vi "Confirm Delays.vi"(3 "Modes":cluster{"A=":u16, "B=":u16, "C=":u16, "D=":u16} {"D=" items=["T0+", "A+", "B+", "C+"]; "C=" items=["T0+", "A+", "B+", "D+"]; "B=" items=["T0+", "A+", "C+", "D+"]; "A=" items=["T0+", "B+", "C+", "D+"]}, 5 "Delays (s)":dbl[](array[numeric]) min=0.0 max=1000.0 format="%#_15f") -> (0 "Modes (out)":cluster{"A=":u16, "B=":u16, "C=":u16, "D=":u16} {"D=" items=["T0+", "A+", "B+", "C+"]; "C=" items=["T0+", "A+", "B+", "D+"]; "B=" items=["T0+", "A+", "C+", "D+"]; "A=" items=["T0+", "B+", "C+", "D+"]}, 2 "Delays (s) (out)":dbl[](array[numeric]) min=0.0 max=1000.0 format="%#_15f")   [LabVIEW 2009]
panel:
  in  "Confirm":bool
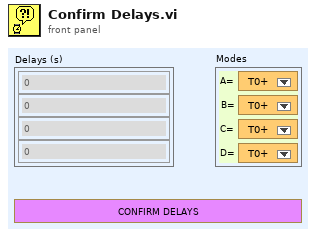
[diagram p1: front panel]
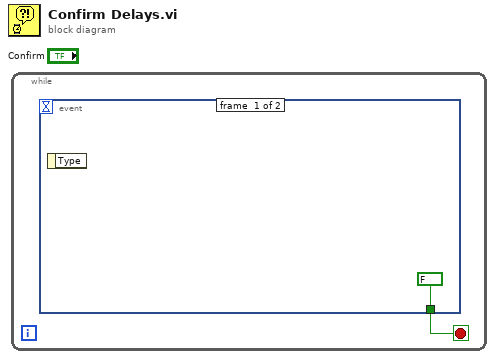
[diagram p0: block diagram]
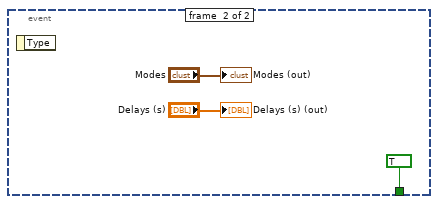
[diagram p2: hidden frame]
diagram:
  n1 = while {
    stop <- w1 stop-if-true
    n2 = event shown="[1] \"Confirm\": Mouse Up" {
      selector: _ -> [_ _]
      dyn-events: _ -> [_ _]
      timeout: _ -> [_ _]
      tunnel: [FALSE TRUE] -> w1
      event #0 {
        n3 = event-data() -> ()  [unwired: 1 in, 1 out]
      }
      event #1 {
        n4 = event-data() -> ()  [unwired: 1 in, 1 out]
        "Delays (s) (out)" <- "Delays (s)"
        "Modes (out)" <- "Modes"
      }
    }
  }
